vi "Get Maximum Data Duration.vi"(11 "variant in":variant) -> (1 "maximum data duration":dbl, 3 "variant out":variant)   [LabVIEW 2017]
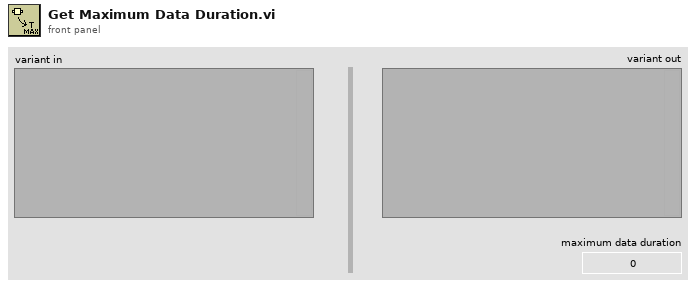
[diagram p1: front panel]
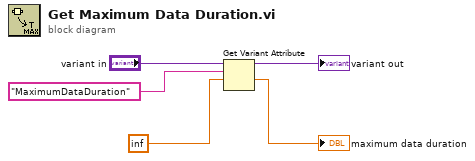
[diagram p0: block diagram]
diagram:
  n1 = Get Variant Attribute(Variant="variant in", name="MaximumDataDuration", default value (empty Variant)=inf ("timestamp")) -> (duplicate Variant=→"variant out":variant, value=→"maximum data duration":dbl)  [unwired: 1 in, 2 out]
